vi "Top Level Init.vi"(8 "error in (no error)":errorcluster, 9 "Node Info":T1, 10 "Core APIs":T2, 11 "Task in":refnum<class "Task.lvclass">) -> (0 "error out":errorcluster, 3 "Task out":refnum<class "Task.lvclass">)   [LabVIEW 2020, in "Volatus.lvlib" / "Task.lvclass"]
uses:
  Task.lvclass
  Core APIs.ctl
  VolatusAPI/VolatusAPI.lvclass
  Node Info.ctl
  Task.lvclass/Task.ctl
  Volatus.lvlib
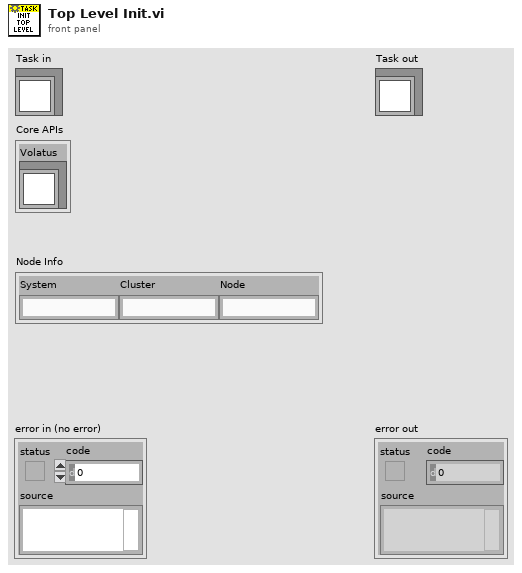
[diagram p1: front panel]
types:
  T1 = typedef "Volatus.lvlib/Task.lvclass/Node Info.ctl" = cluster{"System":string, "Cluster":string, "Node":string}
  T2 = typedef "Volatus.lvlib/Core APIs.ctl" = cluster{"Volatus":refnum<class "VolatusAPI.lvclass">}
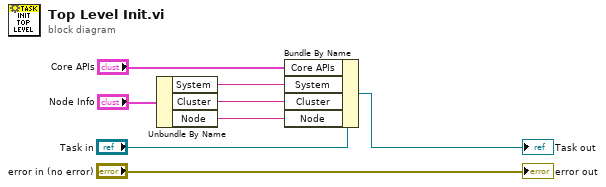
[diagram p0: block diagram]
diagram:
  n1 = Unbundle By Name("Node Info") -> ("System"=w3:string, "Cluster"=w2:string, "Node"=w1:string)
  n2 = Bundle By Name(cluster="Task in", "Core APIs"="Core APIs", "System"=w3, "Cluster"=w2, "Node"=w1) -> (→"Task out":refnum<class "Task.lvclass">)
  "error out" <- "error in (no error)"
